vi "Prepare Control.vi"(7 "VolatusAPI":refnum<class "VolatusAPI.lvclass">, 8 "error in (no error)":errorcluster, 11 "SequencedValves in":refnum<class "SeqDelayControl.lvclass">) -> (0 "error out":errorcluster, 3 "SequencedValves out":refnum<class "SeqDelayControl.lvclass">)   [LabVIEW 2020, in "VolatusControl.lvlib" / "SeqDelayControl.lvclass"]
uses:
  SeqDelayControl.lvclass
  SeqDelayControl.lvclass/SeqDelayControl.ctl
  Volatus/VolatusAPI/VolatusAPI.lvclass
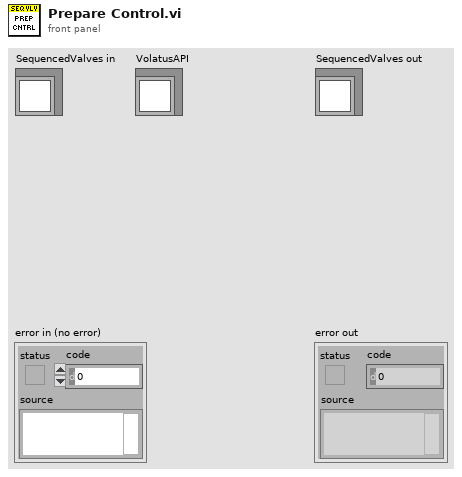
[diagram p1: front panel]
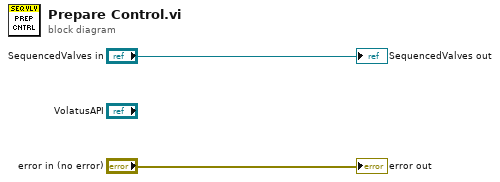
[diagram p0: block diagram]
diagram:
  "error out" <- "error in (no error)"
  "SequencedValves out" <- "SequencedValves in"
